vi "test.vi"() -> ()   [LabVIEW 2018]
panel:
  in  "stop":bool
  in  "x":dbl
  in  "z1":dbl
  in  "z2":dbl
  in  "step":dbl
  in  "speed 1":i32
  in  "speed 2":i32
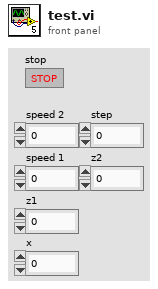
[diagram p1: front panel]
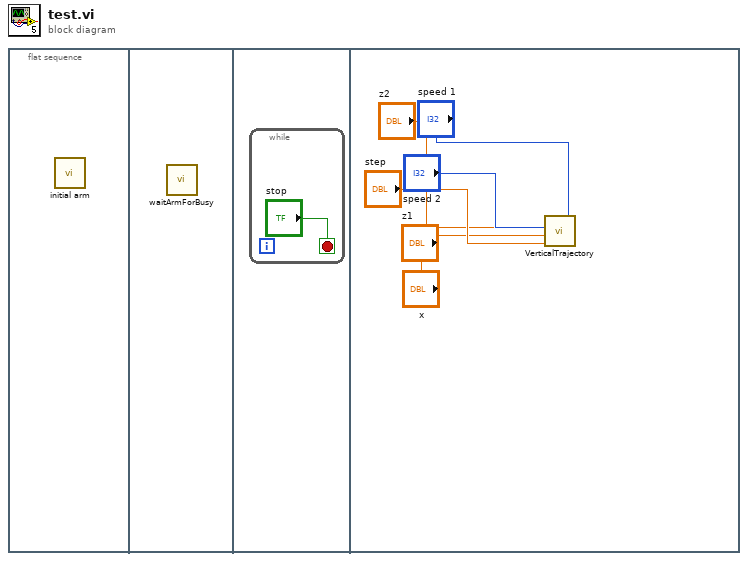
[diagram p0: block diagram]
diagram:
  n1 = flat-sequence {
    frame #0 {
      n2 = call "initial arm.vi"() -> ()  [unwired: 12 in]
    }
    frame #1 {
      n3 = call "waitArmForBusy.vi"() -> ()  [unwired: 12 in]
    }
    frame #2 {
      n4 = while {
        stop <- "stop" stop-if-true
      }
    }
    frame #3 {
      n5 = call "VerticalTrajectory.vi"("speed 2"="speed 2", "speed 1"="speed 1", "step"="step", "z2"="z2", "z1"="z1", "x"="x") -> ()  [unwired: 2 in]
    }
  }
